vi "Route Triggers.vi"(0 "pxi trigger bus configuration [channel]":T2[](array[typedef]), 1 "route for":T3(array[ring]), 2 "map(T)/unmap(F)":bool=TRUE, 5 "direction":T1, 11 "error in":errorcluster) -> (15 "error out":errorcluster)   [LabVIEW 2019]
uses:
  TypeDefs/PXI Trigger Bus Info.ctl
  TypeDefs/Direction.ctl
  <vilib>/Instr/_visa.llb/VISA Unmap Trigger Trigger Source.ctl
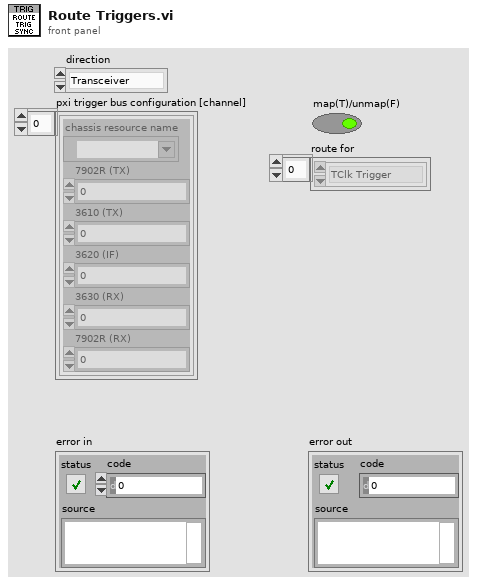
[diagram p1: front panel]
types:
  T1 = typedef "Direction.ctl" = enum16{"Transceiver", "Receiver", "Transmitter"}
  T2 = typedef "PXI Trigger Bus Info.ctl" = cluster{"chassis resource name":refnum<visa-resource-name>, "7902R (TX)":i16, "3610 (TX)":i16, "3620 (IF)":i16, "3630 (RX)":i16, "7902R (RX)":i16}
  T3 = enum16{"TClk Trigger", "TClk Measure", "ADC Sync Injection", "Tx JESD Sync", "Rx JESD Sync", "Tx ADC Sync Injection", "Tx Master10k_Reset"}[]
  T4 = typedef "VISA Unmap Trigger Trigger Source.ctl" = i16
  T5 = cluster{"chassis":refnum<visa-resource-name>, "pxi trigger number":T4, "source trigger segment":i16, "destination trigger segment":i16}
  T6 = cluster{"chassis":refnum<visa-resource-name>, "pxi trigger number":T4, "source trigger segment":i16, "destination trigger segment":i16}[]
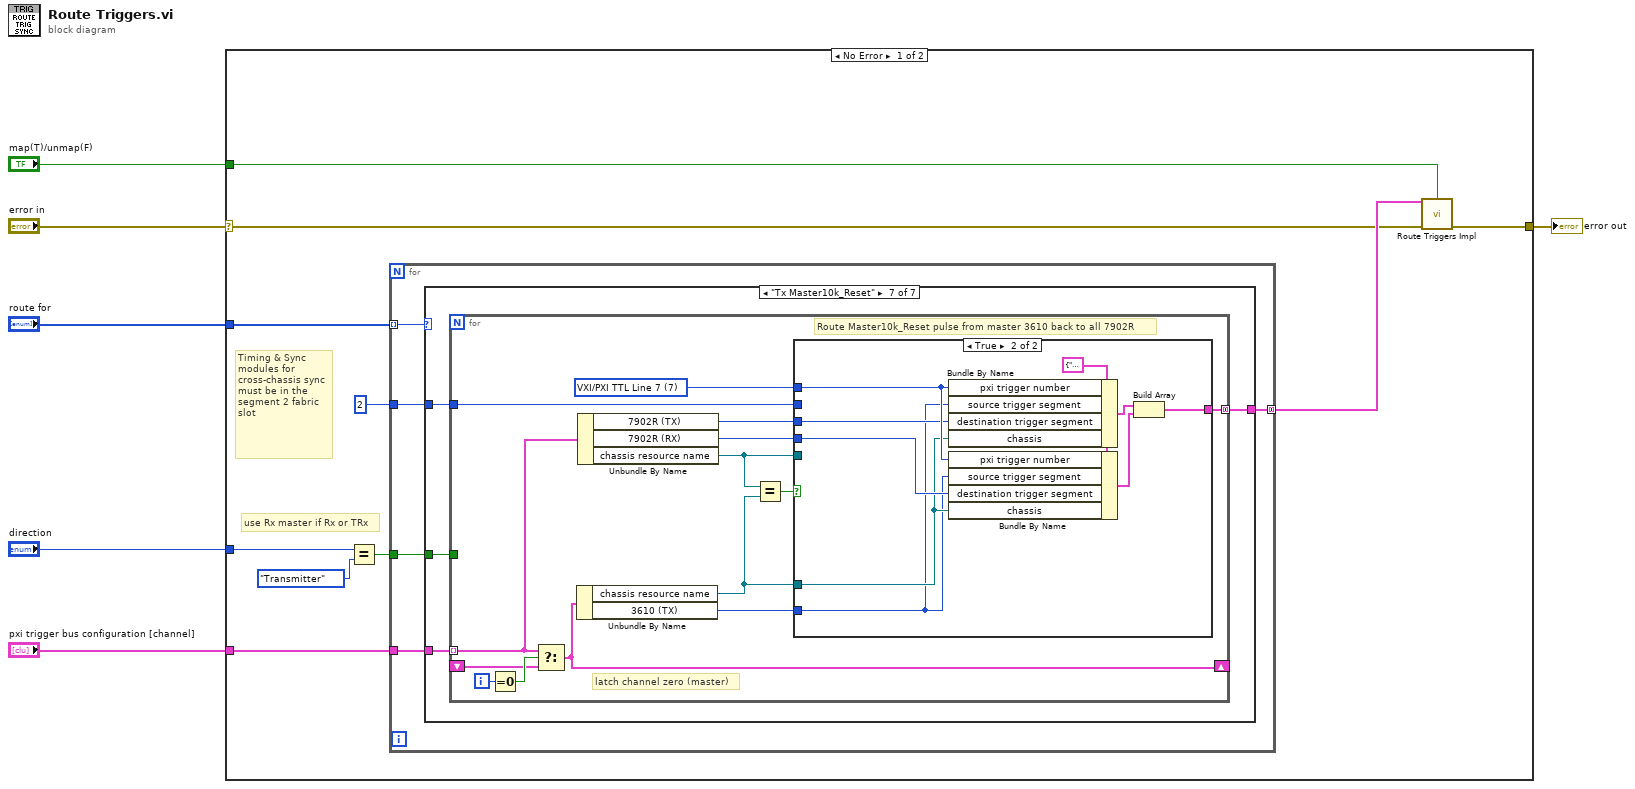
[diagram p0: block diagram]
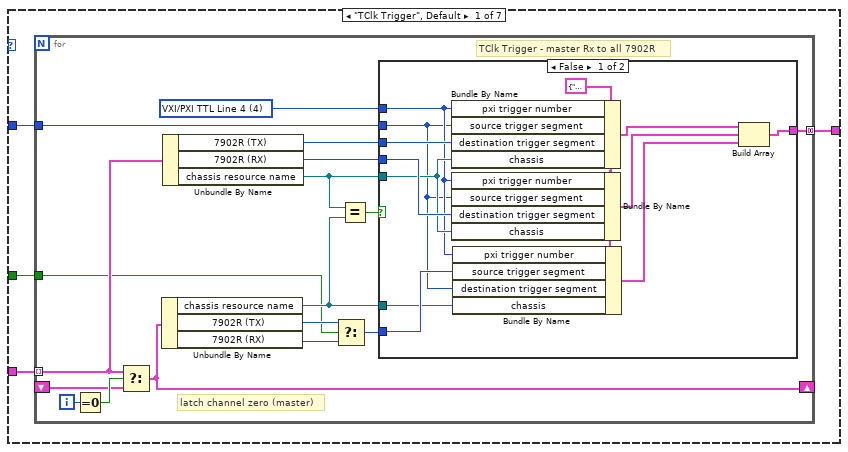
[diagram p2: hidden frame]
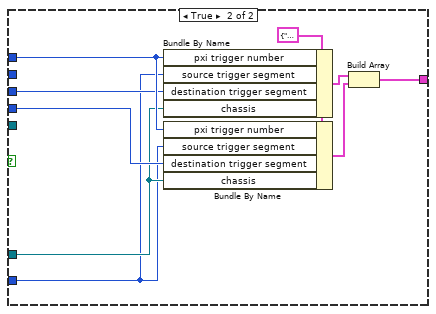
[diagram p3: hidden frame]
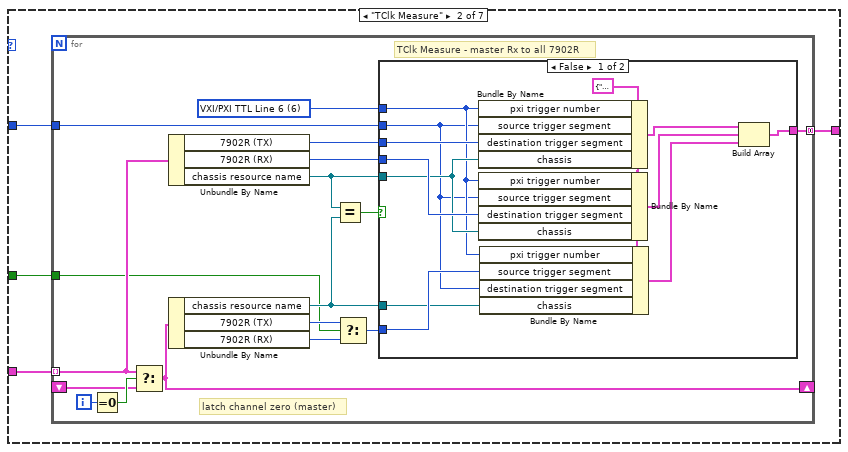
[diagram p4: hidden frame]
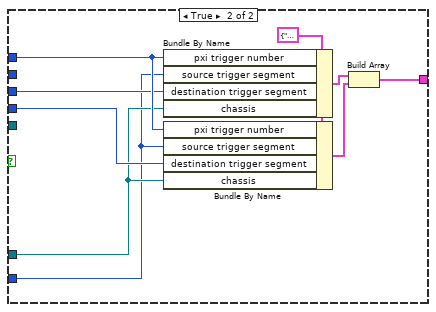
[diagram p5: hidden frame]
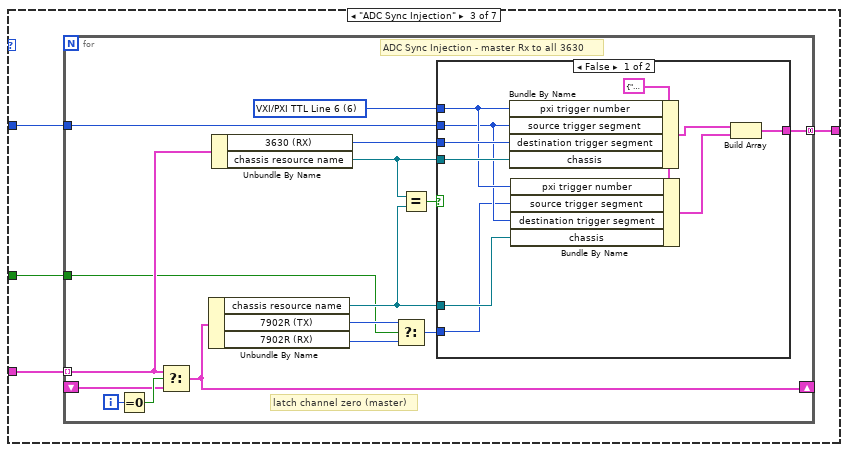
[diagram p6: hidden frame]
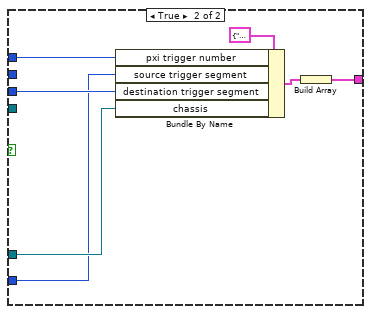
[diagram p7: hidden frame]
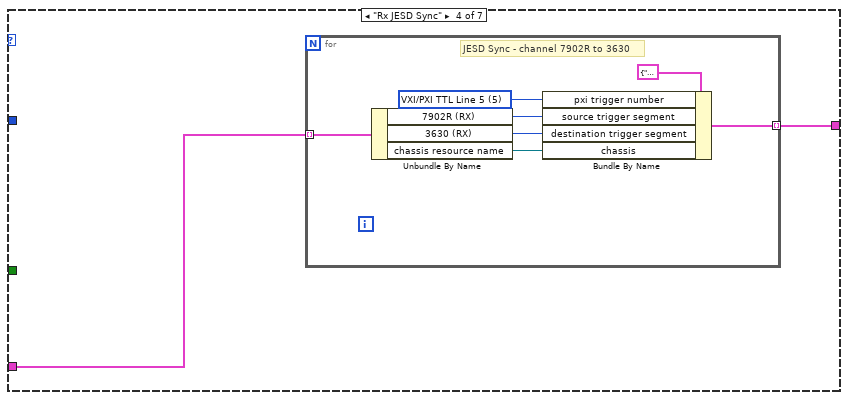
[diagram p8: hidden frame]
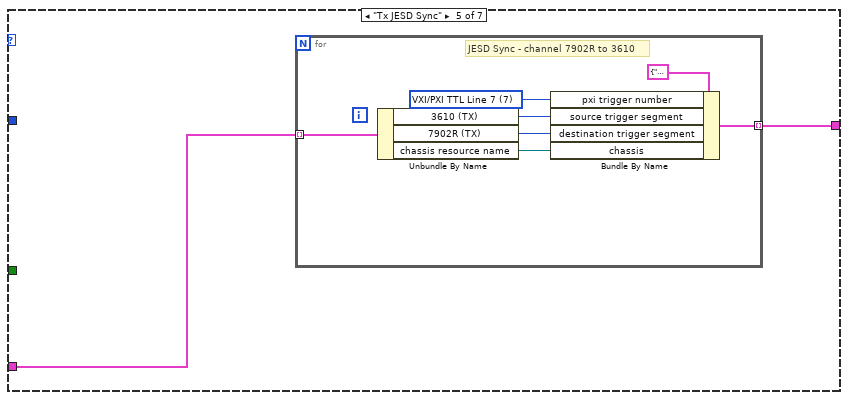
[diagram p9: hidden frame]
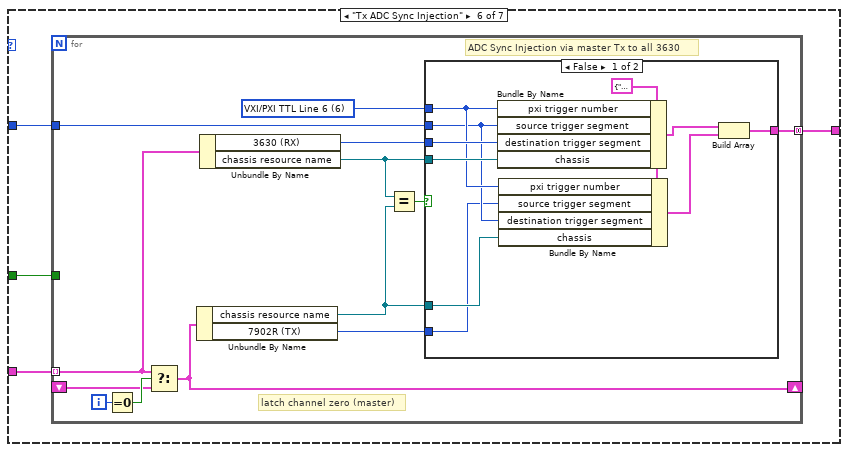
[diagram p10: hidden frame]
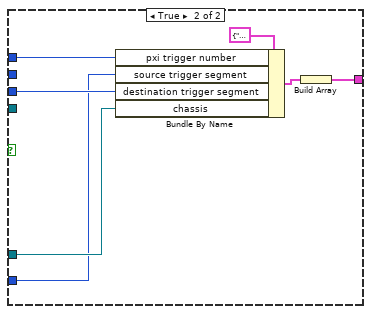
[diagram p11: hidden frame]
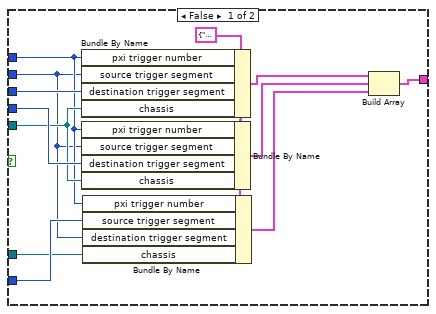
[diagram p12: hidden frame]
diagram:
  n1 = case shown="No Error" "error in" {
    selector: "error in" -> [w9 w234]
    tunnel: [w7 w234] -> w6
    tunnel: "map(T)/unmap(F)" -> [w8 _]
    tunnel: "pxi trigger bus configuration [channel]" -> [w16 _]
    tunnel: "route for" -> [w15 _]
    tunnel: "direction" -> [w11 _]
    frame No Error {
      # "Timing & Sync modules for cross-chassis sync must be in the segment 2 fabric slot"
      # "use Rx master if Rx or TRx"
      n2 = Equal?(x=w11, y=Direction."Transmitter") -> (x = y?=w12:bool)
      n3 = for {
        tunnel: w15 -> [w21] mode=indexing
        tunnel: w16 -> [w20]
        tunnel: [w19] -> w10 mode=concatenating
        tunnel: i16 2 ("source trigger segment") -> [w18]
        tunnel: w12 -> [w17]
        n4 = case shown="\"Tx Master10k_Reset\"" w21 {
          tunnel: w20 -> [w25 w67 w109 w144 w153 w164 w198]
          tunnel: [w24 w66 w108 w143 w152 w161 w197] -> w19
          tunnel: w18 -> [w23 w65 w107 _ _ w162 w196]
          tunnel: w17 -> [w22 w64 w106 _ _ w163 w195]
          frame "TClk Trigger", Default {
            n5 = for {
              tunnel: w25 -> [w36] mode=indexing
              tunnel: [w39] -> w24 mode=concatenating
              shift-right: [w34] -> _
              shift-left: _ -> [w35]
              tunnel: w23 -> [w30]
              tunnel: w22 -> [w26]
              i -> [w42]
              w41 = T4 4 items=["VXI/PXI TTL Line 0"=0, "VXI/PXI TTL Line 1"=1, "VXI/PXI TTL Line 2"=2, "VXI/PXI TTL Line 3"=3, "VXI/PXI TTL Line 4"=4, "VXI/PXI TTL Line 5"=5, "VXI/PXI TTL Line 6"=6, "VXI/PXI TTL Line 7"=7, "VXI ECL Line 0"=8, "VXI ECL Line 1"=9, "Front Panel Input"=27, "Front Panel Output"=28] ("pxi trigger number")
              # "latch channel zero (master)"
              # "TClk Trigger - master Rx to all 7902R"
              n6 = Equal To 0?(x=w42) -> (x = 0?=w38:bool)
              n7 = Select(t=w36, s=w38, f=w35) -> (s? t:f=w34:T2)
              n8 = Unbundle By Name(w34) -> ("chassis resource name"=w33:refnum<visa-resource-name>, "7902R (TX)"=w28:i16, "7902R (RX)"=w27:i16)
              n9 = Unbundle By Name(w36) -> ("7902R (TX)"=w37:i16, "7902R (RX)"=w40:i16, "chassis resource name"=w31:refnum<visa-resource-name>)
              n10 = Select(t=w28, s=w26, f=w27) -> (s? t:f=w29:i16)
              n11 = Equal?(x=w31, y=w33) -> (x = y?=w32:bool)
              n12 = case shown="False" w32 {
                tunnel: w41 -> [w47 w63]
                tunnel: w40 -> [w54 w62]
                tunnel: [w51 w59] -> w39
                tunnel: w37 -> [w50 w57]
                tunnel: w33 -> [w45 w56]
                tunnel: w29 -> [w46 w55]
                tunnel: w30 -> [w43 _]
                tunnel: w31 -> [w49 _]
                frame False {
                  w48 = T5 {"chassis"="", "pxi trigger number"=0, "source trigger segment"=0, "destination trigger segment"=0} ("Trigger Route")
                  n13 = Bundle By Name(cluster=w48, "pxi trigger number"=w47, "source trigger segment"=w43, "destination trigger segment"=w50, "chassis"=w49) -> (w53:T5)
                  n14 = Bundle By Name(cluster=w48, "pxi trigger number"=w47, "source trigger segment"=w43, "destination trigger segment"=w54, "chassis"=w49) -> (w52:T5)
                  n15 = Bundle By Name(cluster=w48, "pxi trigger number"=w47, "source trigger segment"=w46, "destination trigger segment"=w43, "chassis"=w45) -> (w44:T5)
                  n16 = Build Array(w53, w52, w44) -> (w51:T6)
                }
                frame True {
                  w58 = T5 {"chassis"="", "pxi trigger number"=0, "source trigger segment"=0, "destination trigger segment"=0} ("Trigger Route")
                  n17 = Bundle By Name(cluster=w58, "pxi trigger number"=w63, "source trigger segment"=w55, "destination trigger segment"=w57, "chassis"=w56) -> (w61:T5)
                  n18 = Bundle By Name(cluster=w58, "pxi trigger number"=w63, "source trigger segment"=w55, "destination trigger segment"=w62, "chassis"=w56) -> (w60:T5)
                  n19 = Build Array(w61, w60) -> (w59:T6)
                }
              }
            }
          }
          frame "TClk Measure" {
            n20 = for {
              tunnel: w67 -> [w73] mode=indexing
              tunnel: [w81] -> w66 mode=concatenating
              shift-right: [w77] -> _
              shift-left: _ -> [w78]
              tunnel: w65 -> [w72]
              tunnel: w64 -> [w68]
              i -> [w84]
              w83 = T4 6 items=["VXI/PXI TTL Line 0"=0, "VXI/PXI TTL Line 1"=1, "VXI/PXI TTL Line 2"=2, "VXI/PXI TTL Line 3"=3, "VXI/PXI TTL Line 4"=4, "VXI/PXI TTL Line 5"=5, "VXI/PXI TTL Line 6"=6, "VXI/PXI TTL Line 7"=7, "VXI ECL Line 0"=8, "VXI ECL Line 1"=9, "Front Panel Input"=27, "Front Panel Output"=28] ("pxi trigger number")
              # "TClk Measure - master Rx to all 7902R"
              # "latch channel zero (master)"
              n21 = Equal To 0?(x=w84) -> (x = 0?=w80:bool)
              n22 = Select(t=w73, s=w80, f=w78) -> (s? t:f=w77:T2)
              n23 = Unbundle By Name(w73) -> ("7902R (TX)"=w79:i16, "7902R (RX)"=w82:i16, "chassis resource name"=w74:refnum<visa-resource-name>)
              n24 = Unbundle By Name(w77) -> ("chassis resource name"=w76:refnum<visa-resource-name>, "7902R (TX)"=w69:i16, "7902R (RX)"=w70:i16)
              n25 = Equal?(x=w74, y=w76) -> (x = y?=w75:bool)
              n26 = Select(t=w69, s=w68, f=w70) -> (s? t:f=w71:i16)
              n27 = case shown="False" w75 {
                tunnel: w83 -> [w89 w105]
                tunnel: w82 -> [w96 w104]
                tunnel: [w93 w101] -> w81
                tunnel: w79 -> [w92 w99]
                tunnel: w76 -> [w87 w98]
                tunnel: w71 -> [w88 w97]
                tunnel: w74 -> [w91 _]
                tunnel: w72 -> [w85 _]
                frame False {
                  w90 = T5 {"chassis"="", "pxi trigger number"=0, "source trigger segment"=0, "destination trigger segment"=0} ("Trigger Route")
                  n28 = Bundle By Name(cluster=w90, "pxi trigger number"=w89, "source trigger segment"=w85, "destination trigger segment"=w92, "chassis"=w91) -> (w95:T5)
                  n29 = Bundle By Name(cluster=w90, "pxi trigger number"=w89, "source trigger segment"=w85, "destination trigger segment"=w96, "chassis"=w91) -> (w94:T5)
                  n30 = Bundle By Name(cluster=w90, "pxi trigger number"=w89, "source trigger segment"=w88, "destination trigger segment"=w85, "chassis"=w87) -> (w86:T5)
                  n31 = Build Array(w95, w94, w86) -> (w93:T6)
                }
                frame True {
                  w100 = T5 {"chassis"="", "pxi trigger number"=0, "source trigger segment"=0, "destination trigger segment"=0} ("Trigger Route")
                  n32 = Bundle By Name(cluster=w100, "pxi trigger number"=w105, "source trigger segment"=w97, "destination trigger segment"=w99, "chassis"=w98) -> (w103:T5)
                  n33 = Bundle By Name(cluster=w100, "pxi trigger number"=w105, "source trigger segment"=w97, "destination trigger segment"=w104, "chassis"=w98) -> (w102:T5)
                  n34 = Build Array(w103, w102) -> (w101:T6)
                }
              }
            }
          }
          frame "ADC Sync Injection" {
            n35 = for {
              tunnel: w109 -> [w120] mode=indexing
              tunnel: [w123] -> w108 mode=concatenating
              shift-right: [w118] -> _
              shift-left: _ -> [w119]
              tunnel: w107 -> [w114]
              tunnel: w106 -> [w110]
              i -> [w125]
              w124 = T4 6 items=["VXI/PXI TTL Line 0"=0, "VXI/PXI TTL Line 1"=1, "VXI/PXI TTL Line 2"=2, "VXI/PXI TTL Line 3"=3, "VXI/PXI TTL Line 4"=4, "VXI/PXI TTL Line 5"=5, "VXI/PXI TTL Line 6"=6, "VXI/PXI TTL Line 7"=7, "VXI ECL Line 0"=8, "VXI ECL Line 1"=9, "Front Panel Input"=27, "Front Panel Output"=28] ("pxi trigger number")
              # "ADC Sync Injection - master Rx to all 3630"
              # "latch channel zero (master)"
              n36 = Equal To 0?(x=w125) -> (x = 0?=w122:bool)
              n37 = Select(t=w120, s=w122, f=w119) -> (s? t:f=w118:T2)
              n38 = Unbundle By Name(w118) -> ("chassis resource name"=w117:refnum<visa-resource-name>, "7902R (TX)"=w113:i16, "7902R (RX)"=w112:i16)
              n39 = Unbundle By Name(w120) -> ("3630 (RX)"=w121:i16, "chassis resource name"=w115:refnum<visa-resource-name>)
              n40 = Select(t=w113, s=w110, f=w112) -> (s? t:f=w111:i16)
              n41 = Equal?(x=w115, y=w117) -> (x = y?=w116:bool)
              n42 = case shown="False" w116 {
                tunnel: w124 -> [w130 w142]
                tunnel: [w134 w140] -> w123
                tunnel: w121 -> [w133 w138]
                tunnel: w117 -> [w129 w137]
                tunnel: w115 -> [w132 _]
                tunnel: w114 -> [w127 _]
                tunnel: w111 -> [w126 w136]
                frame False {
                  w131 = T5 {"chassis"="", "pxi trigger number"=0, "source trigger segment"=0, "destination trigger segment"=0} ("Trigger Route")
                  n43 = Bundle By Name(cluster=w131, "pxi trigger number"=w130, "source trigger segment"=w127, "destination trigger segment"=w133, "chassis"=w132) -> (w135:T5)
                  n44 = Bundle By Name(cluster=w131, "pxi trigger number"=w130, "source trigger segment"=w126, "destination trigger segment"=w127, "chassis"=w129) -> (w128:T5)
                  n45 = Build Array(w135, w128) -> (w134:T6)
                }
                frame True {
                  n46 = Bundle By Name(cluster=T5 {"chassis"="", "pxi trigger number"=0, "source trigger segment"=0, "destination trigger segment"=0} ("Trigger Route"), "pxi trigger number"=w142, "source trigger segment"=w136, "destination trigger segment"=w138, "chassis"=w137) -> (w141:T5)
                  n47 = Build Array(w141) -> (w140:T6)
                }
              }
            }
          }
          frame "Rx JESD Sync" {
            n48 = for {
              tunnel: w144 -> [w148] mode=indexing
              tunnel: [w147] -> w143 mode=indexing
              w151 = T4 5 items=["VXI/PXI TTL Line 0"=0, "VXI/PXI TTL Line 1"=1, "VXI/PXI TTL Line 2"=2, "VXI/PXI TTL Line 3"=3, "VXI/PXI TTL Line 4"=4, "VXI/PXI TTL Line 5"=5, "VXI/PXI TTL Line 6"=6, "VXI/PXI TTL Line 7"=7, "VXI ECL Line 0"=8, "VXI ECL Line 1"=9, "Front Panel Input"=27, "Front Panel Output"=28] ("pxi trigger number")
              # "JESD Sync - channel 7902R to 3630"
              n49 = Unbundle By Name(w148) -> ("7902R (RX)"=w149:i16, "3630 (RX)"=w150:i16, "chassis resource name"=w145:refnum<visa-resource-name>)
              n50 = Bundle By Name(cluster=T5 {"chassis"="", "pxi trigger number"=0, "source trigger segment"=0, "destination trigger segment"=0} ("Trigger Route"), "pxi trigger number"=w151, "source trigger segment"=w149, "destination trigger segment"=w150, "chassis"=w145) -> (w147:T5)
            }
          }
          frame "Tx JESD Sync" {
            n51 = for {
              tunnel: w153 -> [w157] mode=indexing
              tunnel: [w156] -> w152 mode=indexing
              w158 = T4 7 items=["VXI/PXI TTL Line 0"=0, "VXI/PXI TTL Line 1"=1, "VXI/PXI TTL Line 2"=2, "VXI/PXI TTL Line 3"=3, "VXI/PXI TTL Line 4"=4, "VXI/PXI TTL Line 5"=5, "VXI/PXI TTL Line 6"=6, "VXI/PXI TTL Line 7"=7, "VXI ECL Line 0"=8, "VXI ECL Line 1"=9, "Front Panel Input"=27, "Front Panel Output"=28] ("pxi trigger number")
              # "JESD Sync - channel 7902R to 3610"
              n52 = Unbundle By Name(w157) -> ("3610 (TX)"=w160:i16, "7902R (TX)"=w159:i16, "chassis resource name"=w154:refnum<visa-resource-name>)
              n53 = Bundle By Name(cluster=T5 {"chassis"="", "pxi trigger number"=0, "source trigger segment"=0, "destination trigger segment"=0} ("Trigger Route"), "pxi trigger number"=w158, "source trigger segment"=w160, "destination trigger segment"=w159, "chassis"=w154) -> (w156:T5)
            }
          }
          frame "Tx ADC Sync Injection" {
            n54 = for {
              tunnel: w164 -> [w172] mode=indexing
              tunnel: [w175] -> w161 mode=concatenating
              shift-right: [w170] -> _
              shift-left: _ -> [w171]
              tunnel: w162 -> [w166]
              tunnel: w163 -> [_]
              i -> [w177]
              w176 = T4 6 items=["VXI/PXI TTL Line 0"=0, "VXI/PXI TTL Line 1"=1, "VXI/PXI TTL Line 2"=2, "VXI/PXI TTL Line 3"=3, "VXI/PXI TTL Line 4"=4, "VXI/PXI TTL Line 5"=5, "VXI/PXI TTL Line 6"=6, "VXI/PXI TTL Line 7"=7, "VXI ECL Line 0"=8, "VXI ECL Line 1"=9, "Front Panel Input"=27, "Front Panel Output"=28] ("pxi trigger number")
              # "ADC Sync Injection via master Tx to all 3630"
              # "latch channel zero (master)"
              n55 = Equal To 0?(x=w177) -> (x = 0?=w174:bool)
              n56 = Select(t=w172, s=w174, f=w171) -> (s? t:f=w170:T2)
              n57 = Unbundle By Name(w170) -> ("chassis resource name"=w169:refnum<visa-resource-name>, "7902R (TX)"=w165:i16)
              n58 = Unbundle By Name(w172) -> ("3630 (RX)"=w173:i16, "chassis resource name"=w167:refnum<visa-resource-name>)
              n59 = Equal?(x=w167, y=w169) -> (x = y?=w168:bool)
              n60 = case shown="False" w168 {
                tunnel: w176 -> [w182 w194]
                tunnel: [w186 w192] -> w175
                tunnel: w173 -> [w185 w190]
                tunnel: w169 -> [w181 w189]
                tunnel: w167 -> [w184 _]
                tunnel: w166 -> [w179 _]
                tunnel: w165 -> [w178 w188]
                frame False {
                  w183 = T5 {"chassis"="", "pxi trigger number"=0, "source trigger segment"=0, "destination trigger segment"=0} ("Trigger Route")
                  n61 = Bundle By Name(cluster=w183, "pxi trigger number"=w182, "source trigger segment"=w179, "destination trigger segment"=w185, "chassis"=w184) -> (w187:T5)
                  n62 = Bundle By Name(cluster=w183, "pxi trigger number"=w182, "source trigger segment"=w178, "destination trigger segment"=w179, "chassis"=w181) -> (w180:T5)
                  n63 = Build Array(w187, w180) -> (w186:T6)
                }
                frame True {
                  n64 = Bundle By Name(cluster=T5 {"chassis"="", "pxi trigger number"=0, "source trigger segment"=0, "destination trigger segment"=0} ("Trigger Route"), "pxi trigger number"=w194, "source trigger segment"=w188, "destination trigger segment"=w190, "chassis"=w189) -> (w193:T5)
                  n65 = Build Array(w193) -> (w192:T6)
                }
              }
            }
          }
          frame "Tx Master10k_Reset" {
            n66 = for {
              tunnel: w198 -> [w206] mode=indexing
              tunnel: [w209] -> w197 mode=concatenating
              shift-right: [w204] -> _
              shift-left: _ -> [w205]
              tunnel: w196 -> [w200]
              tunnel: w195 -> [_]
              i -> [w212]
              w211 = T4 7 items=["VXI/PXI TTL Line 0"=0, "VXI/PXI TTL Line 1"=1, "VXI/PXI TTL Line 2"=2, "VXI/PXI TTL Line 3"=3, "VXI/PXI TTL Line 4"=4, "VXI/PXI TTL Line 5"=5, "VXI/PXI TTL Line 6"=6, "VXI/PXI TTL Line 7"=7, "VXI ECL Line 0"=8, "VXI ECL Line 1"=9, "Front Panel Input"=27, "Front Panel Output"=28] ("pxi trigger number")
              # "latch channel zero (master)"
              # "Route Master10k_Reset pulse from master 3610 back to all 7902R"
              n67 = Equal To 0?(x=w212) -> (x = 0?=w208:bool)
              n68 = Select(t=w206, s=w208, f=w205) -> (s? t:f=w204:T2)
              n69 = Unbundle By Name(w204) -> ("chassis resource name"=w203:refnum<visa-resource-name>, "3610 (TX)"=w199:i16)
              n70 = Unbundle By Name(w206) -> ("7902R (TX)"=w207:i16, "7902R (RX)"=w210:i16, "chassis resource name"=w201:refnum<visa-resource-name>)
              n71 = Equal?(x=w201, y=w203) -> (x = y?=w202:bool)
              n72 = case shown="True" w202 {
                tunnel: w211 -> [w217 w233]
                tunnel: w210 -> [w224 w232]
                tunnel: [w221 w229] -> w209
                tunnel: w207 -> [w220 w227]
                tunnel: w203 -> [w215 w226]
                tunnel: w199 -> [w216 w225]
                tunnel: w200 -> [w213 _]
                tunnel: w201 -> [w219 _]
                frame False {
                  w218 = T5 {"chassis"="", "pxi trigger number"=0, "source trigger segment"=0, "destination trigger segment"=0} ("Trigger Route")
                  n73 = Bundle By Name(cluster=w218, "pxi trigger number"=w217, "source trigger segment"=w213, "destination trigger segment"=w220, "chassis"=w219) -> (w223:T5)
                  n74 = Bundle By Name(cluster=w218, "pxi trigger number"=w217, "source trigger segment"=w213, "destination trigger segment"=w224, "chassis"=w219) -> (w222:T5)
                  n75 = Bundle By Name(cluster=w218, "pxi trigger number"=w217, "source trigger segment"=w216, "destination trigger segment"=w213, "chassis"=w215) -> (w214:T5)
                  n76 = Build Array(w223, w222, w214) -> (w221:T6)
                }
                frame True {
                  w228 = T5 {"chassis"="", "pxi trigger number"=0, "source trigger segment"=0, "destination trigger segment"=0} ("Trigger Route")
                  n77 = Bundle By Name(cluster=w228, "pxi trigger number"=w233, "source trigger segment"=w225, "destination trigger segment"=w227, "chassis"=w226) -> (w231:T5)
                  n78 = Bundle By Name(cluster=w228, "pxi trigger number"=w233, "source trigger segment"=w225, "destination trigger segment"=w232, "chassis"=w226) -> (w230:T5)
                  n79 = Build Array(w231, w230) -> (w229:T6)
                }
              }
            }
          }
        }
      }
      n80 = call "Route Triggers Impl.vi"("trigger routes"=w10, "map(T)/unmap(F)"=w8, "error in"=w9) -> ("error out"=w7:errorcluster)  [unwired: 12 in]
    }
    frame Error {
    }
  }
  "error out" <- w6
